vi "Resolve Entry.vi"(8 "error in (no error)":errorcluster, 11 "Test Run Request":refnum<class "Test Run Request.lvclass">) -> (0 "error out":errorcluster, 3 "Entry":string)   [LabVIEW 2026, in "Generic Execution Adapter.lvclass"]
uses:
  Generic Execution Adapter.lvclass
  Generic Execution Adapter.lvclass/Generic Execution Adapter.ctl
  Domain/Test Run Request/Test Run Request.lvclass
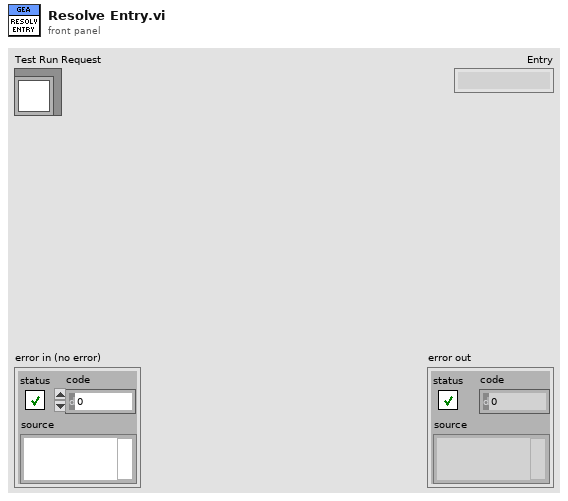
[diagram p1: front panel]
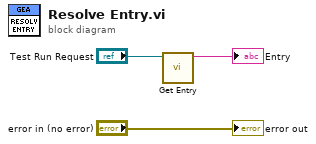
[diagram p0: block diagram]
diagram:
  n1 = call "Get Entry.vi"("Test Run Request"="Test Run Request") -> ("Entry"=→"Entry":string)  [unwired: 10 in]
  "error out" <- "error in (no error)"
